vi "globalTearDown.vi"(8 "error in (no error)":errorcluster, 11 "testcase-CSMManagementAPI in":refnum<class "testcase-CSMManagementAPI.lvclass">) -> (0 "error out":errorcluster, 3 "testcase-CSMManagementAPI out":refnum<class "testcase-CSMManagementAPI.lvclass">)   [LabVIEW 2017, in "testcase-CSMManagementAPI.lvclass"]
uses:
  testcase-CSMManagementAPI.lvclass
  <vilib>/addons/_JKI Toolkits/VI Tester/TestCase.llb/TestCase.lvclass
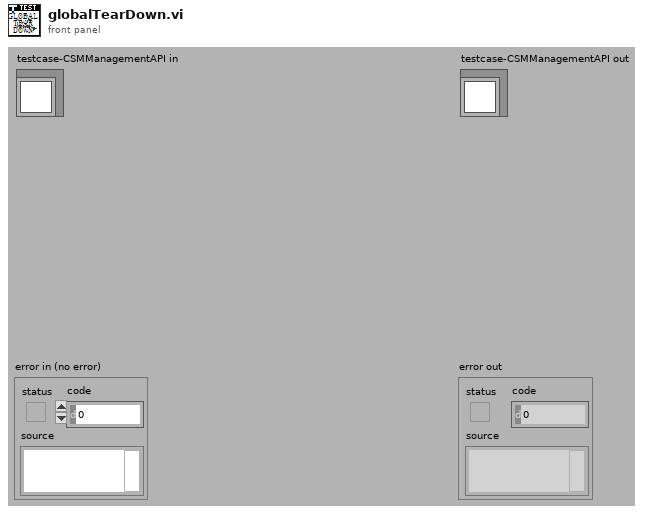
[diagram p1: front panel]
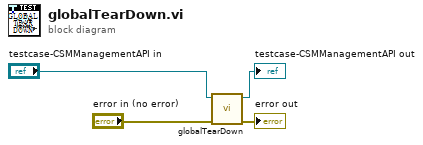
[diagram p0: block diagram]
diagram:
  n1 = call-parent "globalTearDown.vi"("error in (no error)"="error in (no error)", "TestCase in"="testcase-CSMManagementAPI in") -> ("error out"=→"error out":errorcluster, "TestCase out"=→"testcase-CSMManagementAPI out":refnum<class "testcase-CSMManagementAPI.lvclass">)  [unwired: 8 in]
